vi "SetSetpoint2.vi"(8 "Error In":errorcluster, 10 "Setpoint (C)":dbl, 11 "Omega CSi32 In":refnum<visa-resource-name>) -> (0 "Error Out":errorcluster, 3 "Omega CSi32 Out":refnum<visa-resource-name>)   [LabVIEW 2012, in "Omega-CSi32.lvlib"]
uses:
  Omega-CSi32.lvlib
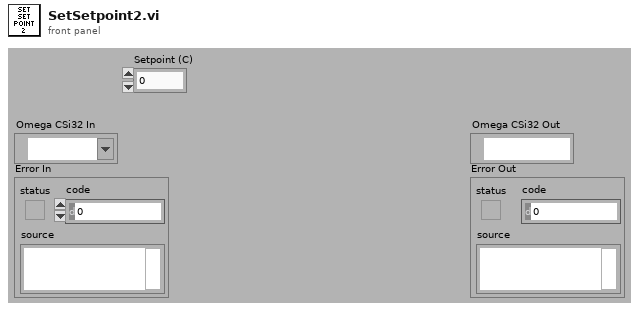
[diagram p1: front panel]
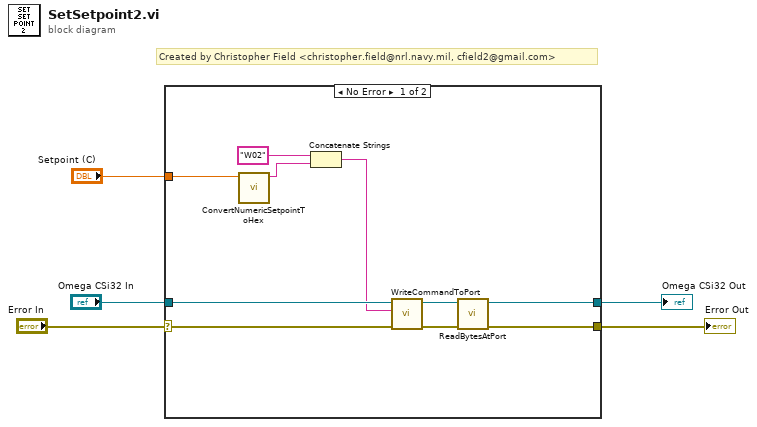
[diagram p0: block diagram]
diagram:
  # "Created by Christopher Field <christopher.field@nrl.navy.mil, cfield2@gmail.com>"
  n1 = case shown="No Error" "Error In" {
    selector: "Error In" -> [w6 w16]
    tunnel: "Setpoint (C)" -> [w15 _]
    tunnel: "Omega CSi32 In" -> [w12 w17]
    tunnel: [w9 w17] -> w3
    tunnel: [w8 w16] -> w2
    frame No Error {
      n2 = call "ConvertNumericSetpointToHex.vi"("Numeric Setpoint (C)"=w15) -> ("Hex Setpoint (C)"=w14:string)  [unwired: 10 in]
      n3 = Concatenate Strings("W02" ("Command"), w14) -> (w11:string)
      n4 = call "WriteCommandToPort.vi"("Error In"=w6, "Command"=w11, "CSi32 In"=w12) -> ("Error Out"=w7:errorcluster, "CSi32 Out"=w10:refnum<visa-resource-name>)  [unwired: 7 in]
      n5 = call "ReadBytesAtPort.vi"("Error In"=w7, "CSi32 In"=w10) -> ("Error Out"=w8:errorcluster, "CSi32 Out"=w9:refnum<visa-resource-name>)  [unwired: 7 in, 1 out]
    }
    frame Error {
    }
  }
  "Omega CSi32 Out" <- w3
  "Error Out" <- w2
